vi "Velocity_FFT.vi"(0 "Sampling Frequency":dbl, 1 "Samples":i32) -> (2 "Peaks":dbl[][](array[numeric]), 3 "t_vect":dbl[](array[numeric]), 4 "error out":errorcluster)   [LabVIEW 2017]
uses:
  <vilib>/Analysis/2dsp.llb/Real FFT.vi
  <vilib>/Analysis/NI_AALPro.lvlib
  <vilib>/ptbypt/NI_PtbyPt.lvlib
  <vilib>/Analysis/NI_AAL_SigProc.lvlib
panel:
  out "XY Graph 2":cluster{"Y":dbl[], "Y":dbl[]}[](graph)
  out "XY Graph":cluster{"Y":dbl[], "Y":dbl[]}[](graph)
  out "Phase":dbl[](array[numeric])
  out "Magnitude":dbl[](array[numeric])
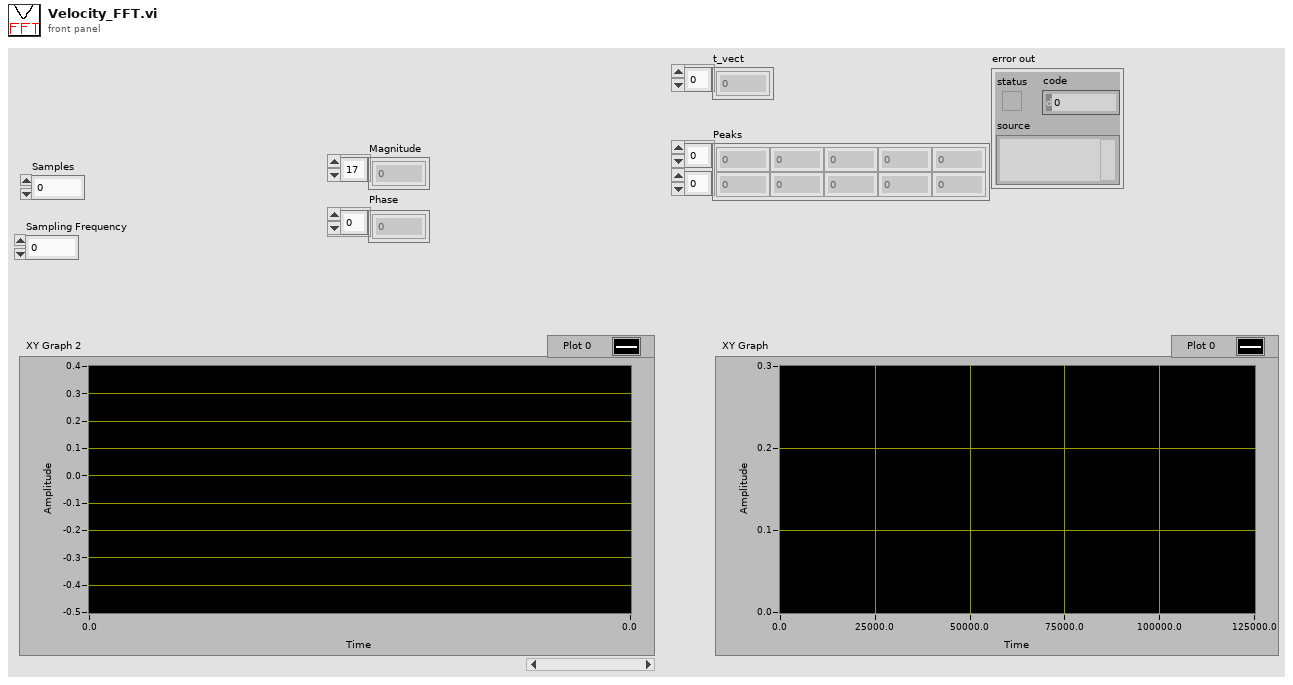
[diagram p1: front panel]
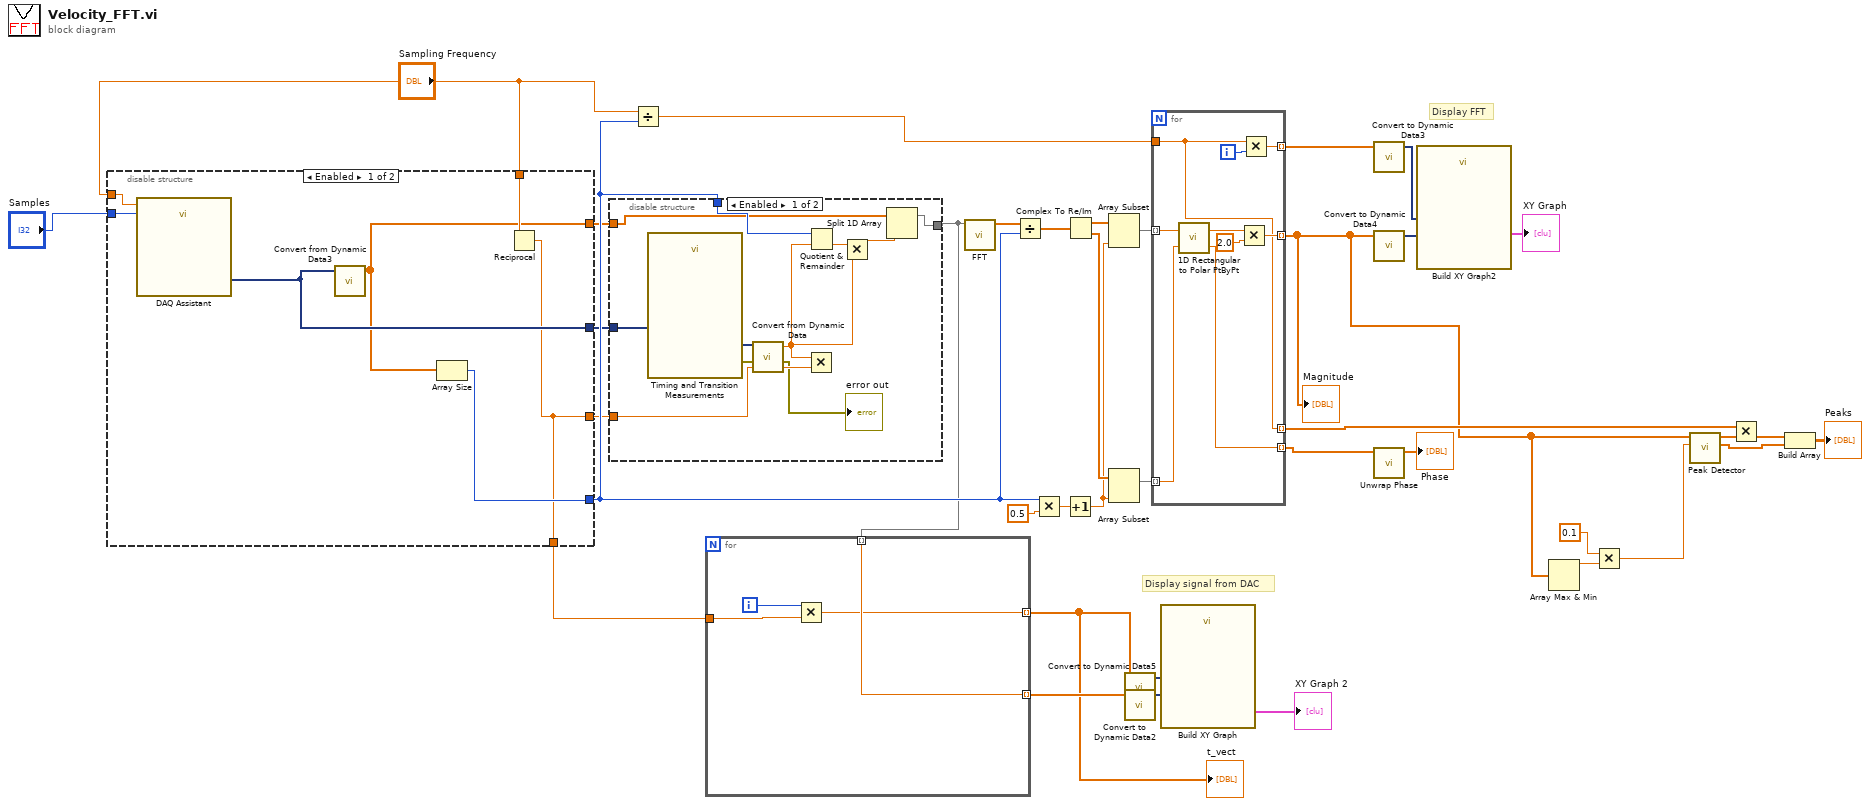
[diagram p0: block diagram]
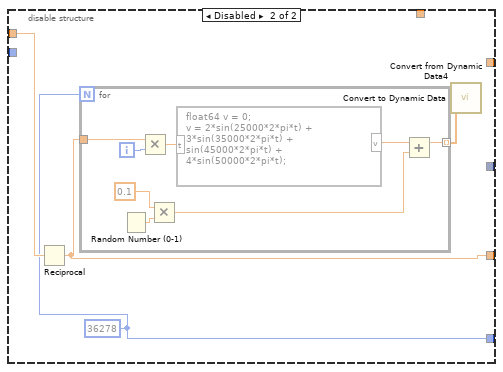
[diagram p3: hidden frame]
diagram:
  # "Display FFT"
  # "Display signal from DAC"
  n1 = disable-structure shown="Enabled" {
    disable-tunnel: "Sampling Frequency" -> [w44 w50]
    disable-tunnel: [w40 w49] -> w4
    disable-tunnel: [w45 w47] -> w13
    disable-tunnel: "Sampling Frequency" -> [w43 _]
    disable-tunnel: [w42 _] -> w10
    disable-tunnel: [w41 _] -> w2
    disable-tunnel: [w40 _] -> w7
    disable-tunnel: "Samples" -> [w39 _]
    frame Enabled {
      n2 = call "DAQ Assistant"("rate"=w44, "number of samples"=w39) -> ("data"=w42:dynamicdata)  [unwired: 15 in, 2 out]
      n3 = call "Convert from Dynamic Data3"("Dynamic Data Type"=w42) -> ("Array"=w41:dbl[])  [unwired: 3 in]
      n4 = Array Size(array=w41) -> (size(s)=w45:i32)
      n5 = Reciprocal(x=w43) -> (1/x=w40:dbl)
    }
    frame Disabled {
      w47 = 36278 ("Samples")
      n6 = Reciprocal(x=w50) -> (1/x=w49:dbl)
      n7 = for {
        N: w47 -> [_]
        tunnel: w49 -> [w58]
        tunnel: [w52] -> w48 mode=indexing
        i -> [w55]
        n8 = Random Number (0-1)() -> (number: 0 to 1=w53:dbl)
        n9 = Multiply(x=w58, y=w55) -> (x*y=w57:dbl)
        n10 = Multiply(x=0.1, y=w53) -> (x*y=w51:dbl)
        n11 = formula code="float64 v = 0;\nv = 2*sin(25000*2*pi*t) +\n3*sin(35000*2*pi*t) +\nsin(45000*2*pi*t) +\n4*sin(50000*2*pi*t);"("t"=w57) -> ("v"=w56:dbl)
        n12 = Add(x=w56, y=w51) -> (x+y=w52:dbl)
      }
      n13 = call "Convert to Dynamic Data"("Array"=w48) -> ("Dynamic Data Type"=w46:dynamicdata)  [unwired: 3 in]
      n14 = call "Convert from Dynamic Data4"("Dynamic Data Type"=w46) -> ()  [unwired: 3 in, 1 out]
    }
  }
  n15 = disable-structure shown="Enabled" {
    disable-tunnel: w13 -> [w66 _]
    disable-tunnel: w10 -> [w65 _]
    disable-tunnel: w4 -> [w63 _]
    disable-tunnel: [w59 w69] -> w1
    disable-tunnel: w2 -> [w61 w69]
    frame Enabled {
      n16 = call "Timing and Transition Measurements"("Signals"=w65) -> ("error out"=→"error out":errorcluster, "Period"=w68:dynamicdata)  [unwired: 9 in]
      n17 = call "Convert from Dynamic Data"("Dynamic Data Type"=w68) -> ("Scalar"=w67:dbl)  [unwired: 3 in]
      n18 = Multiply(x=w67, y=w63) -> ()  [unwired: 1 out]
      n19 = Quotient & Remainder(x=w66, y=w67) -> (floor(x/y)=w64:dbl)  [unwired: 1 out]
      n20 = Multiply(x=w64, y=w67) -> (x*y=w60:dbl)
      n21 = Split 1D Array(array=w61, index=w60) -> (first subarray=w59:dbl[])  [unwired: 1 out]
    }
    frame Disabled {
    }
  }
  n22 = Divide(x="Sampling Frequency", y=w13) -> (x/y=w29:dbl)
  n23 = for {
    tunnel: w1 -> [w73] mode=indexing
    tunnel: [w73] -> w8 mode=indexing
    tunnel: w7 -> [w71]
    tunnel: [w70] -> w3 mode=indexing
    i -> [w72]
    n24 = Multiply(x=w72, y=w71) -> (x*y=w70:dbl)
  }
  "t_vect" <- w3
  n25 = call-poly <vilib>:"FFT.vi"("X"=w1) -> ("FFT {X}"=w23:cdb[])  [unwired: 9 in, 1 out]
  n26 = Divide(x=w23, y=w13) -> (x/y=w32:cdb[])
  n27 = Multiply(x=w13, y=0.5) -> (x*y=w36:dbl)
  n28 = Increment(x=w36) -> (x+1=w25:dbl)
  n29 = Complex To Re/Im(x + iy=w32) -> (x=w38:dbl[], y=w35:dbl[])
  n30 = Array Subset(array=w38, length=w25) -> (w34:dbl[])  [unwired: 1 in]
  n31 = Array Subset(array=w35, length=w25) -> (w33:dbl[])  [unwired: 1 in]
  n32 = call "Convert to Dynamic Data5"("Array"=w3) -> ("Dynamic Data Type"=w6:dynamicdata)  [unwired: 3 in]
  n33 = call "Convert to Dynamic Data2"("Array"=w8) -> ("Dynamic Data Type"=w9:dynamicdata)  [unwired: 3 in]
  n34 = for {
    tunnel: w34 -> [w82] mode=indexing
    tunnel: w33 -> [w81] mode=indexing
    tunnel: [w78] -> w17 mode=indexing
    tunnel: [w77] -> w30 mode=indexing
    tunnel: w29 -> [w74]
    tunnel: [w76] -> w24 mode=indexing
    tunnel: [w74] -> w20 mode=indexing
    i -> [w75]
    n35 = call <vilib>:"1D Rectangular to Polar PtByPt.vi"("y"=w81, "x"=w82) -> ("phase"=w77:dbl, "magnitude"=w80:dbl)
    n36 = Multiply(x=w80, y=2.0) -> (x*y=w78:dbl)
    n37 = Multiply(x=w74, y=w75) -> (x*y=w76:dbl)
  }
  "Magnitude" <- w17
  n38 = call "Build XY Graph"("Y Input"=w9, "X Input"=w6) -> ("XY Graph"=→"XY Graph 2":cluster{"X":dbl[], "Y":dbl[]}[])  [unwired: 8 in, 1 out]
  n39 = call "Convert to Dynamic Data3"("Array"=w24) -> ("Dynamic Data Type"=w27:dynamicdata)  [unwired: 3 in]
  n40 = call "Convert to Dynamic Data4"("Array"=w17) -> ("Dynamic Data Type"=w26:dynamicdata)  [unwired: 3 in]
  n41 = call <vilib>:"Unwrap Phase.vi"("Phase"=w30) -> ("Unwrapped Phase"=→"Phase":dbl[])  [unwired: 9 in, 1 out]
  n42 = call "Build XY Graph2"("Y Input"=w26, "X Input"=w27) -> ("XY Graph"=→"XY Graph":cluster{"X":dbl[], "Y":dbl[]}[])  [unwired: 8 in, 1 out]
  n43 = Array Max & Min(array=w17) -> (max value=w16:dbl)  [unwired: 3 out]
  n44 = Multiply(x=0.1 ("threshold"), y=w16) -> (x*y=w14:dbl)
  n45 = call <vilib>:"Peak Detector.vi"("threshold"=w14, "X"=w17) -> ("Amplitudes"=w19:dbl[], "Locations"=w22:dbl[])  [unwired: 5 in, 3 out]
  n46 = Multiply(x=w20, y=w22) -> (x*y=w21:dbl[])
  n47 = Build Array(w21, w19) -> (→"Peaks":dbl[][])
